vi "Cliente - Fabrica.vi"() -> ()   [LabVIEW 2018]
doc: "Date Client.vi reads the date and time sent from Date Server.vi. The VI first reads 4 bytes defining the length of the date string, then reads the date. Once the stop button is pressed, Date Client sends a single character to tell Date Server to terminate."
uses:
  <vilib>/Utility/file.llb/Write Delimited Spreadsheet (string).vi
panel:
  out "Numeric":dbl
  in  "INICIAR / RESET":bool
  in  "Report:":bool
  in  "RESET \nDE SIMULA敲O":bool
  in  "Emergência":bool
  out "Chave":string
  out "Pedido":string
  out "Pedido":u32(colorbox)
  out "Funcionamento:":string
  out "Funcionamento:":u32(colorbox)
  out "LED Forno":bool
  out "LED Misturador":bool
  out "Protocolo de Comunicação - Produção":string
  out "Estoque \nProduto Final":dbl(slide) scale=0.0..2500.0
  in  "Esteira":bool
  out "Estoque \nForno":dbl(slide) scale=0.0..2000.0
  out "Thermometro\nForno":dbl(slide) scale=0.0..100.0
  in  "Contagem de Estoque OK?":bool
  out "Estoque B utilizado:":dbl
  in  "Estoque A utilizado:":dbl
  out "Estoque \nMisturador":dbl(slide) scale=0.0..2000.0
  in  "Estoque Produto B":dbl min=0.0 max=1000.0
  in  "Estoque Produto A":dbl=1000.0 min=0.0 max=1000.0
  out "Estoque \nProduto B [KG]":dbl(slide) scale=0.0..1200.0
  out "Estoque \nProduto A [KG]":dbl(slide) scale=0.0..1200.0
  out "Protocolo de Ordens de Produção:":string
  in  "Temperatura Desejada Forno °C":dbl(knob) scale=0.0..100.0
  in  "Histórico":i32(listbox)
  out "RESET":dbl
  out "Temperatura Caldeira":dbl
  out "Produto B":dbl
  out "Produto A":dbl
  out "Estado Motor Esteira":dbl
  out "VETOR DE SAIDA":dbl[](array[numeric])
  in  "stop":bool
  out "Mensagem Recebida":string
  in  "Enviar":bool
  in  "Mensagem":string
  in  "Endereço IP":string
  in  "Porta que será utilizada para a conexão":u16=6341
  # "Cliente - Chão de Fábrica"
  # "Comunicação TCP/IP  -  CLIENTE"
  # "Produção Infante Calderaria"
  # "CONTROLE DE ESTOQUE:"
  # "Digite o inventário realizado \ndas matérias - primas abaixo:"
  # "Digite o estoque que será utilizado em produção:"
  # "CONTROLE DE PRODU敲O:"
  # "ORDENS DE PRODU敲O:"
  # "1 - ON ; 0 - OFF"
  # "1 - ON ; 0 - OFF"
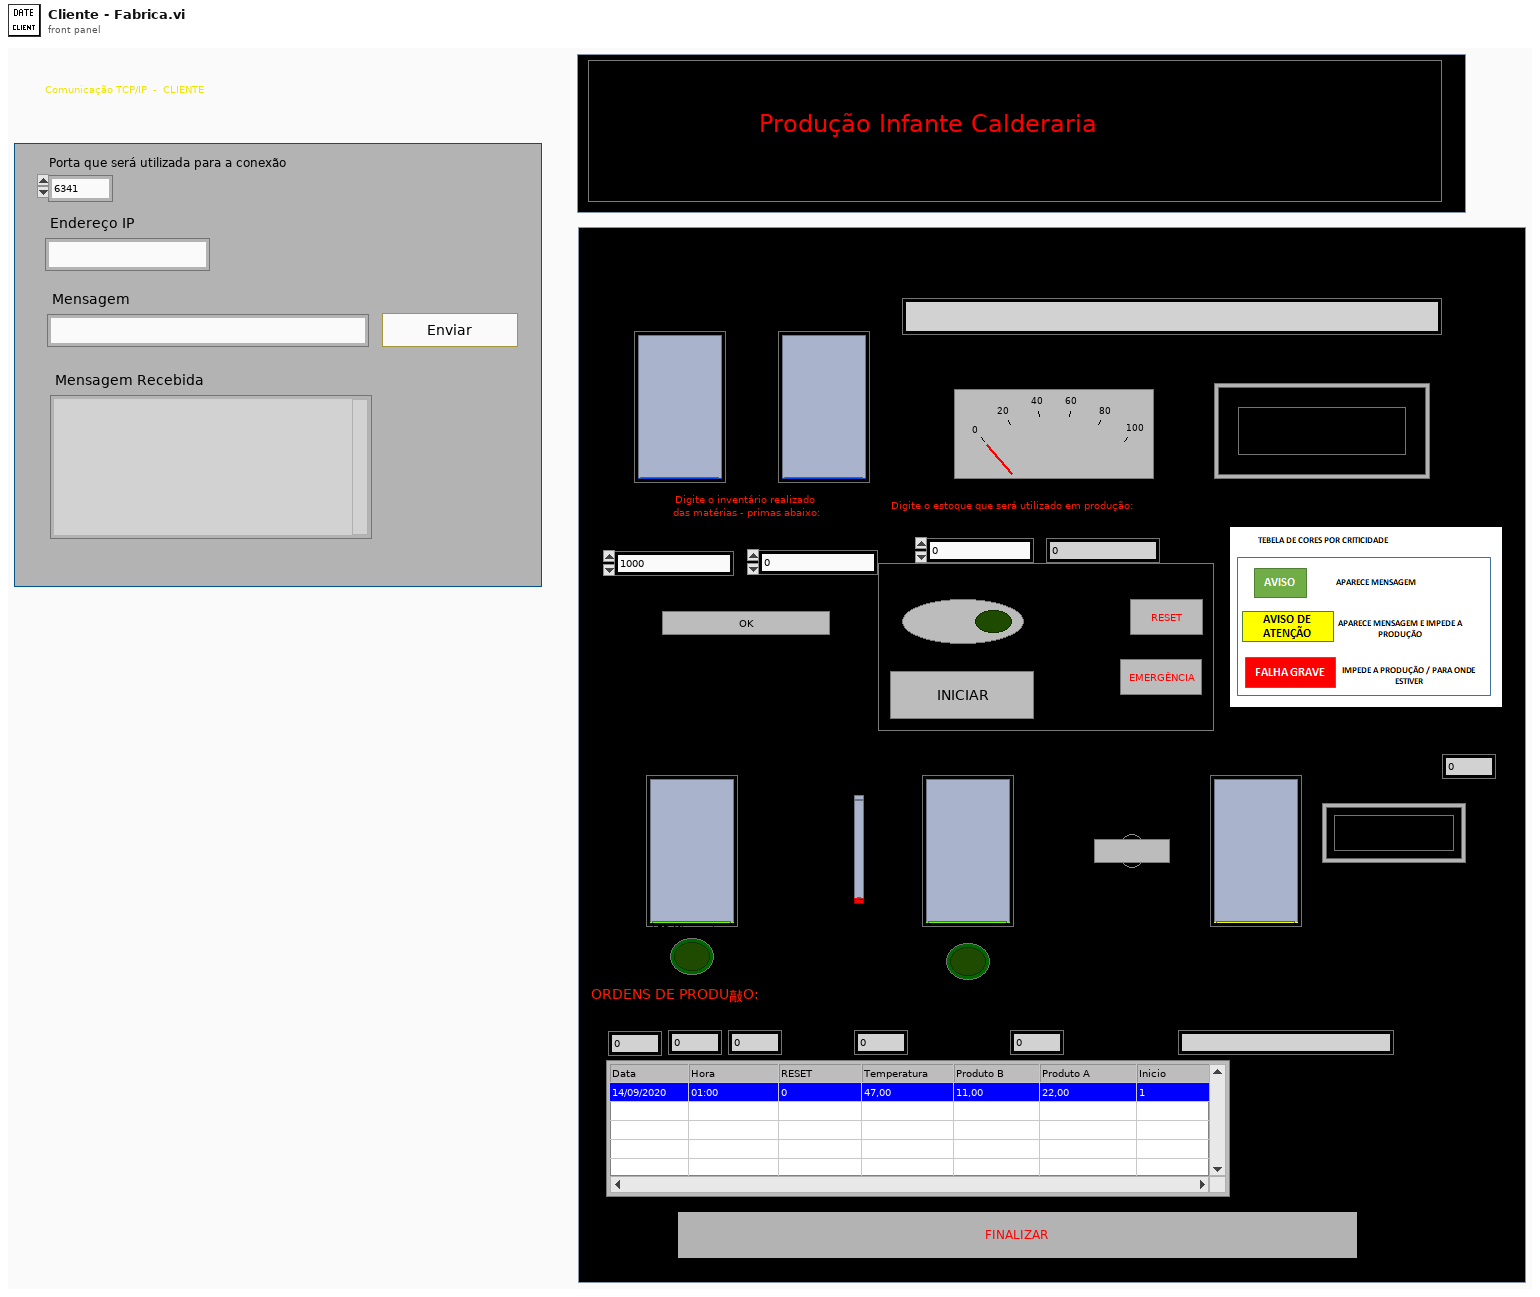
[diagram p1: front panel]
types:
  T1 = enum16{"Standard", "Buffered", "CRLF", "Immediate"}
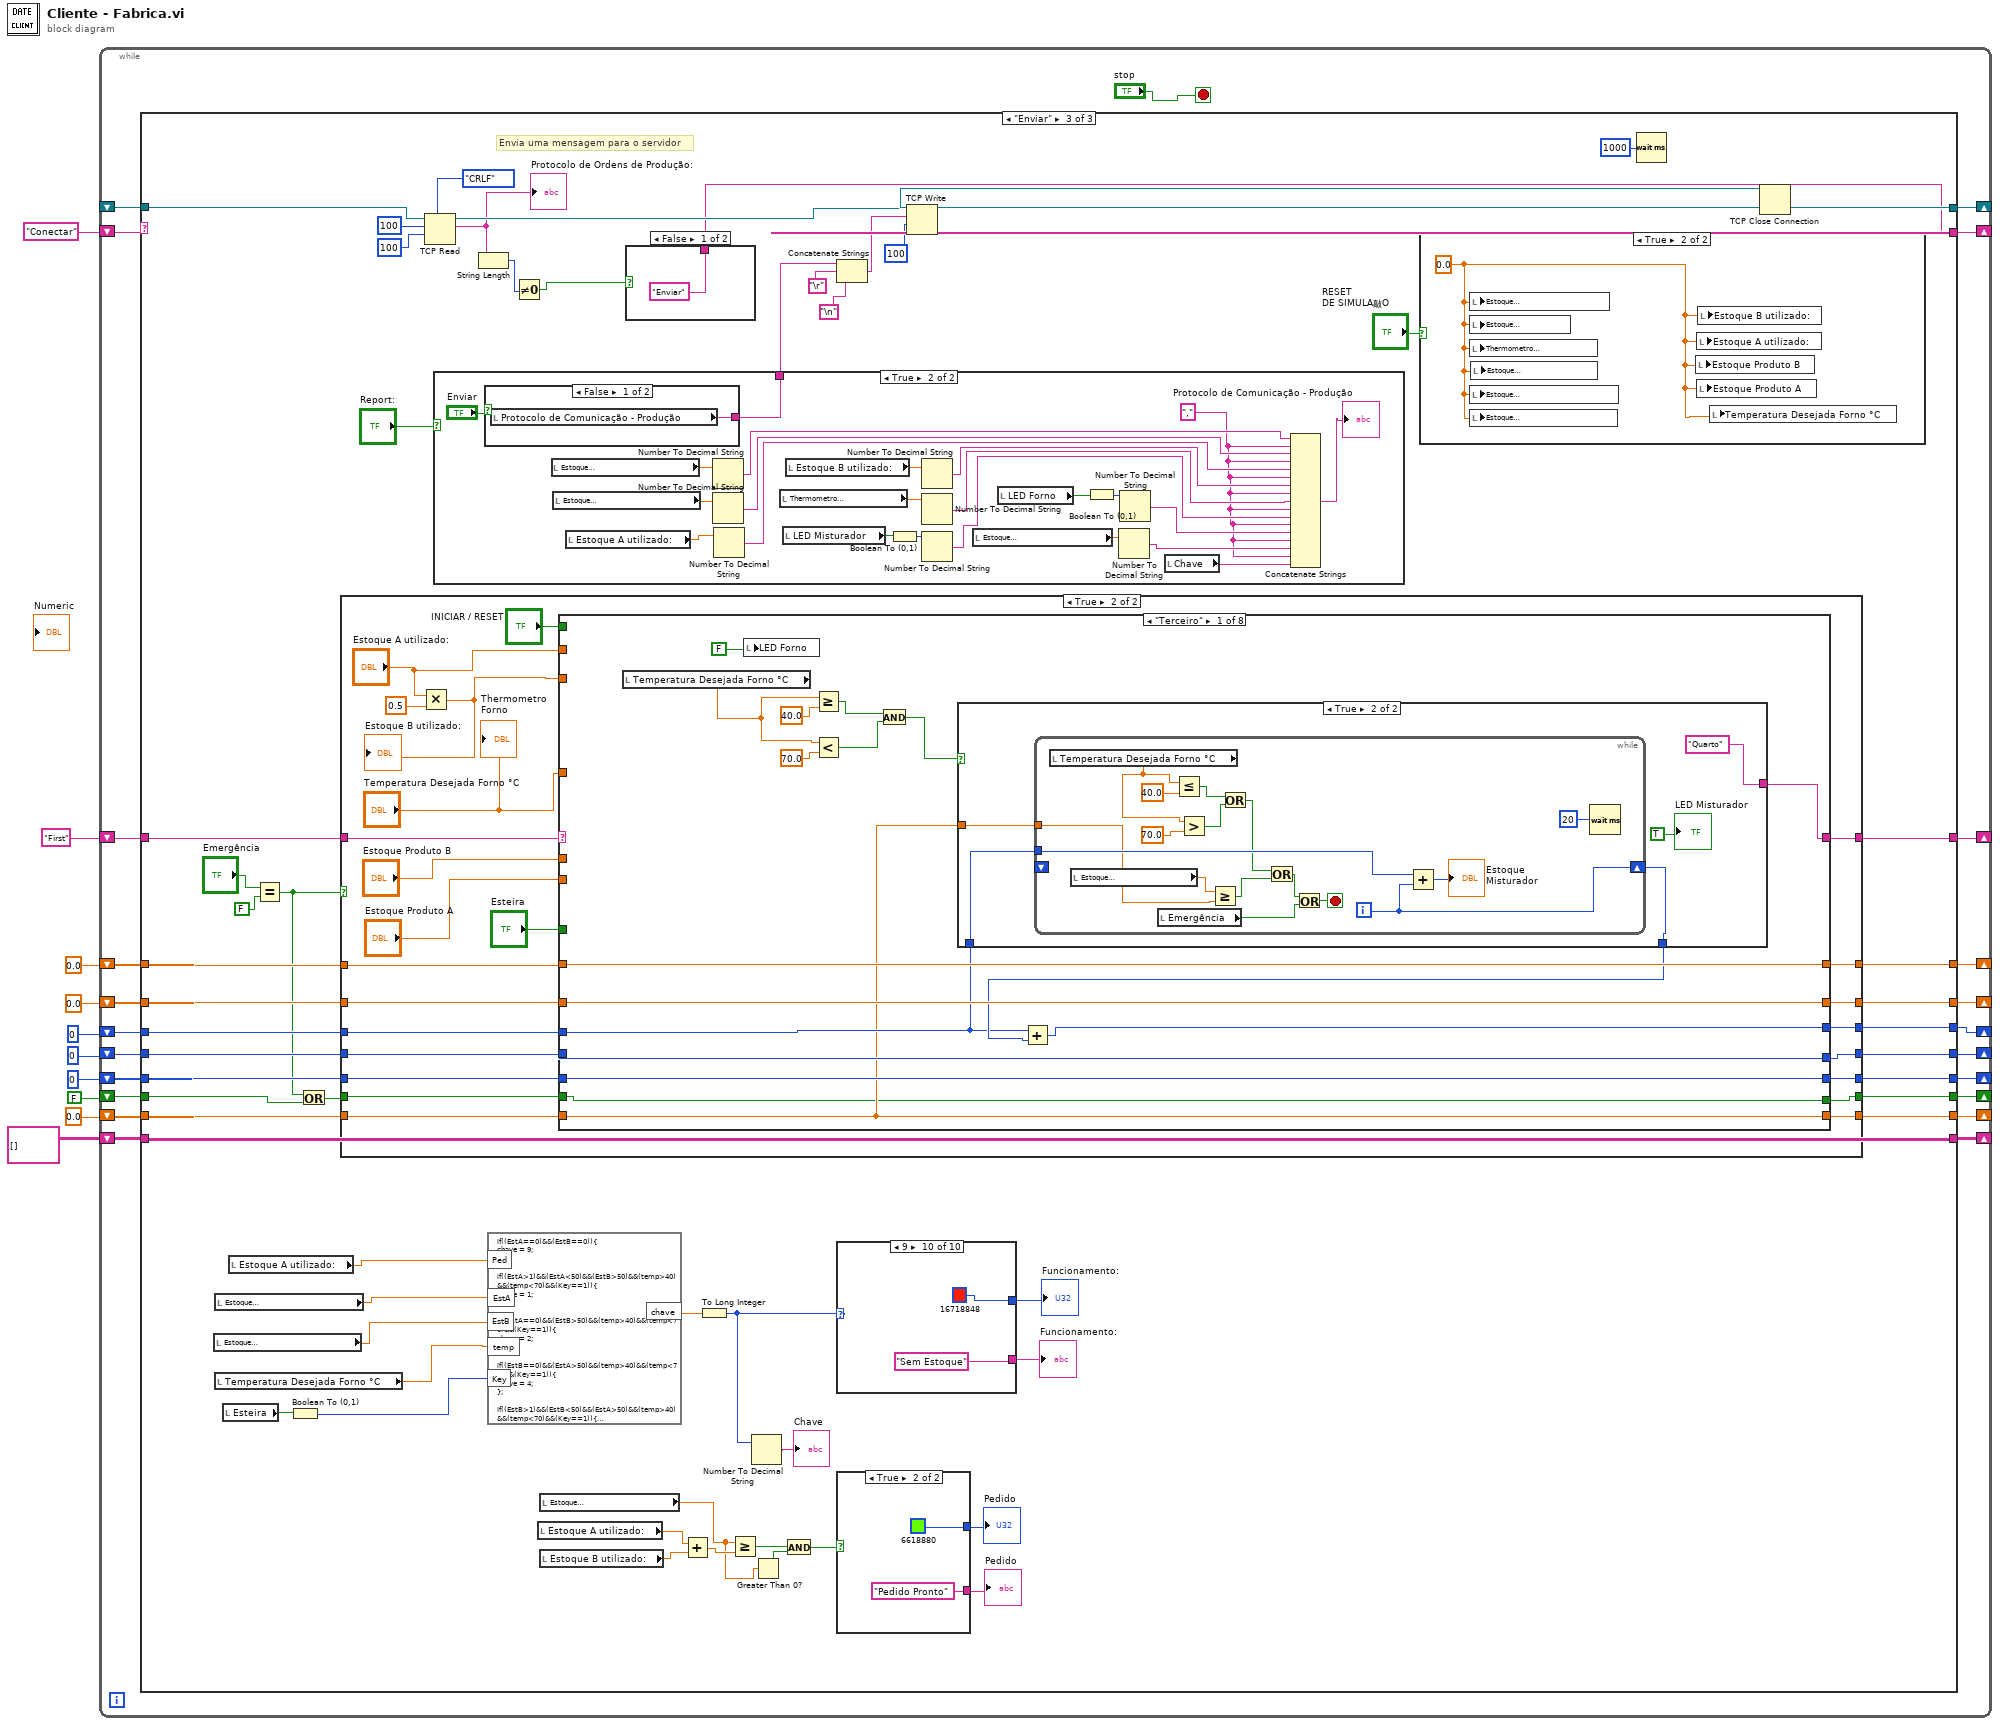
[diagram p0: block diagram]
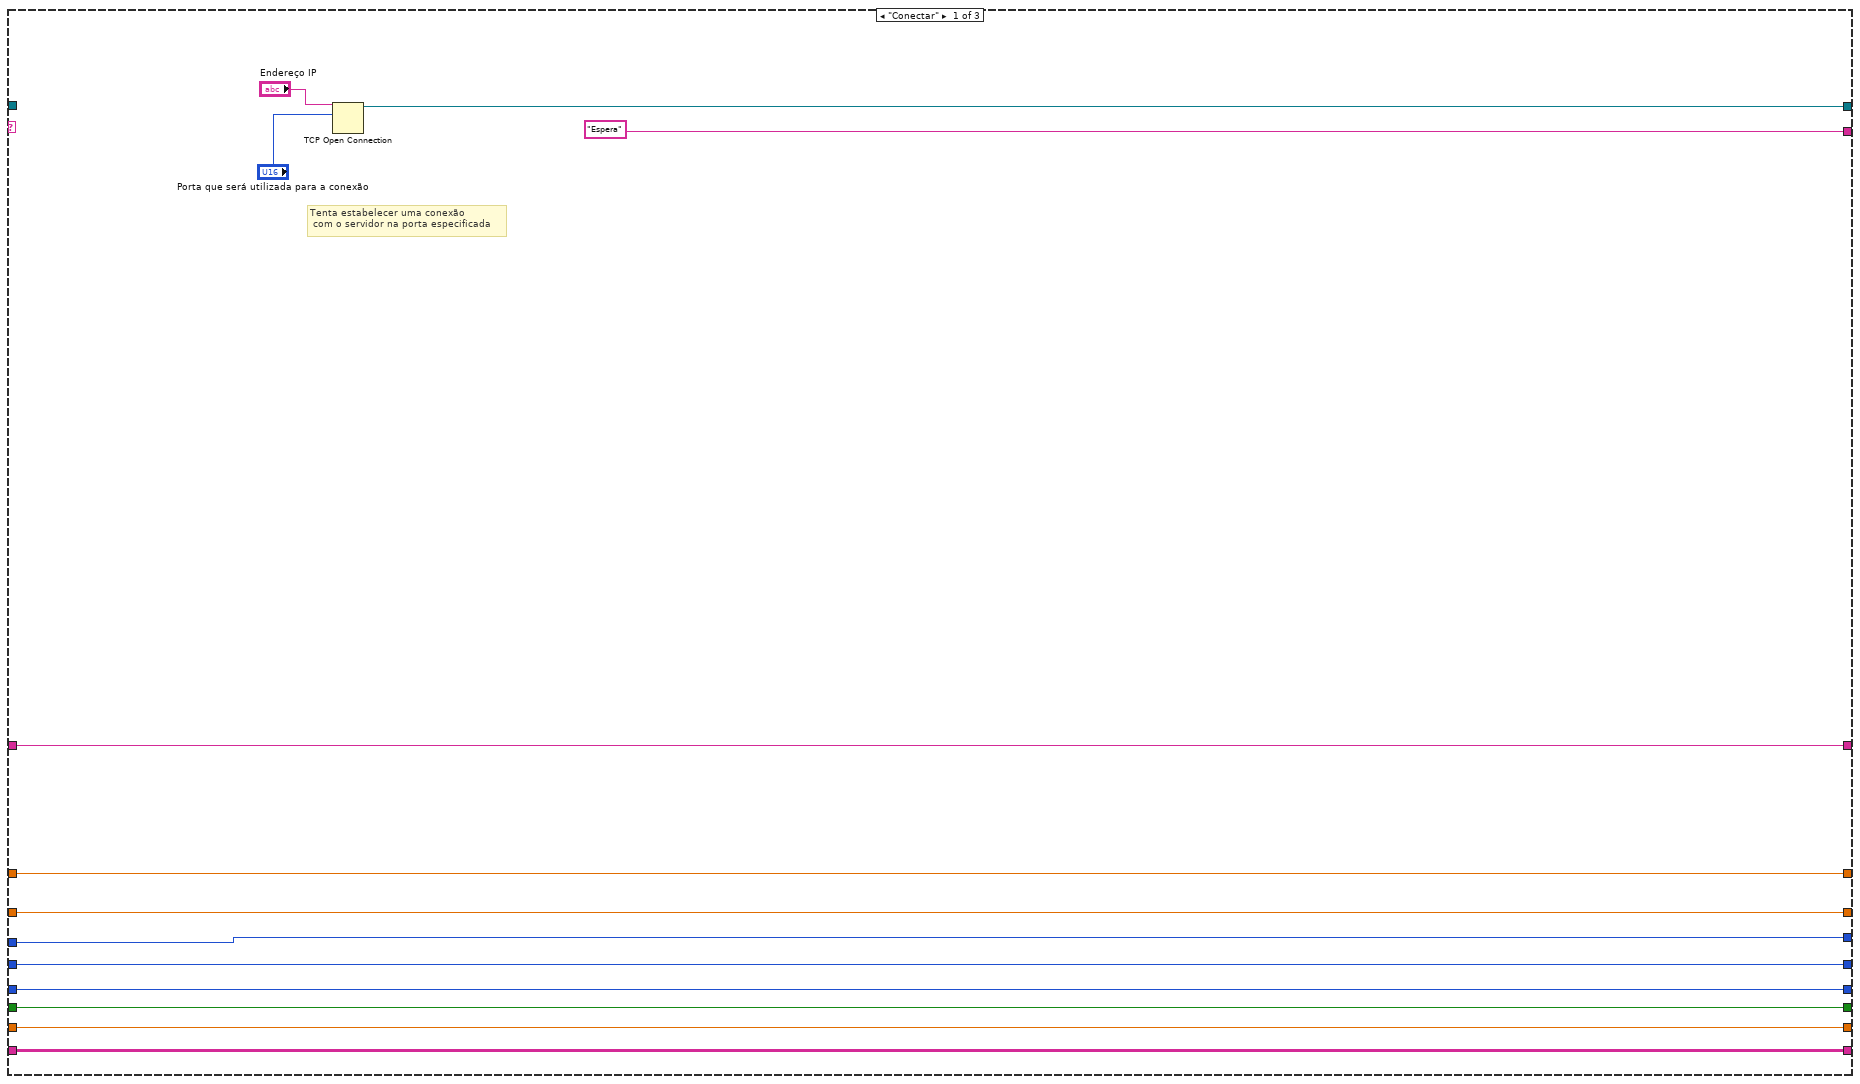
[diagram p2: hidden frame]
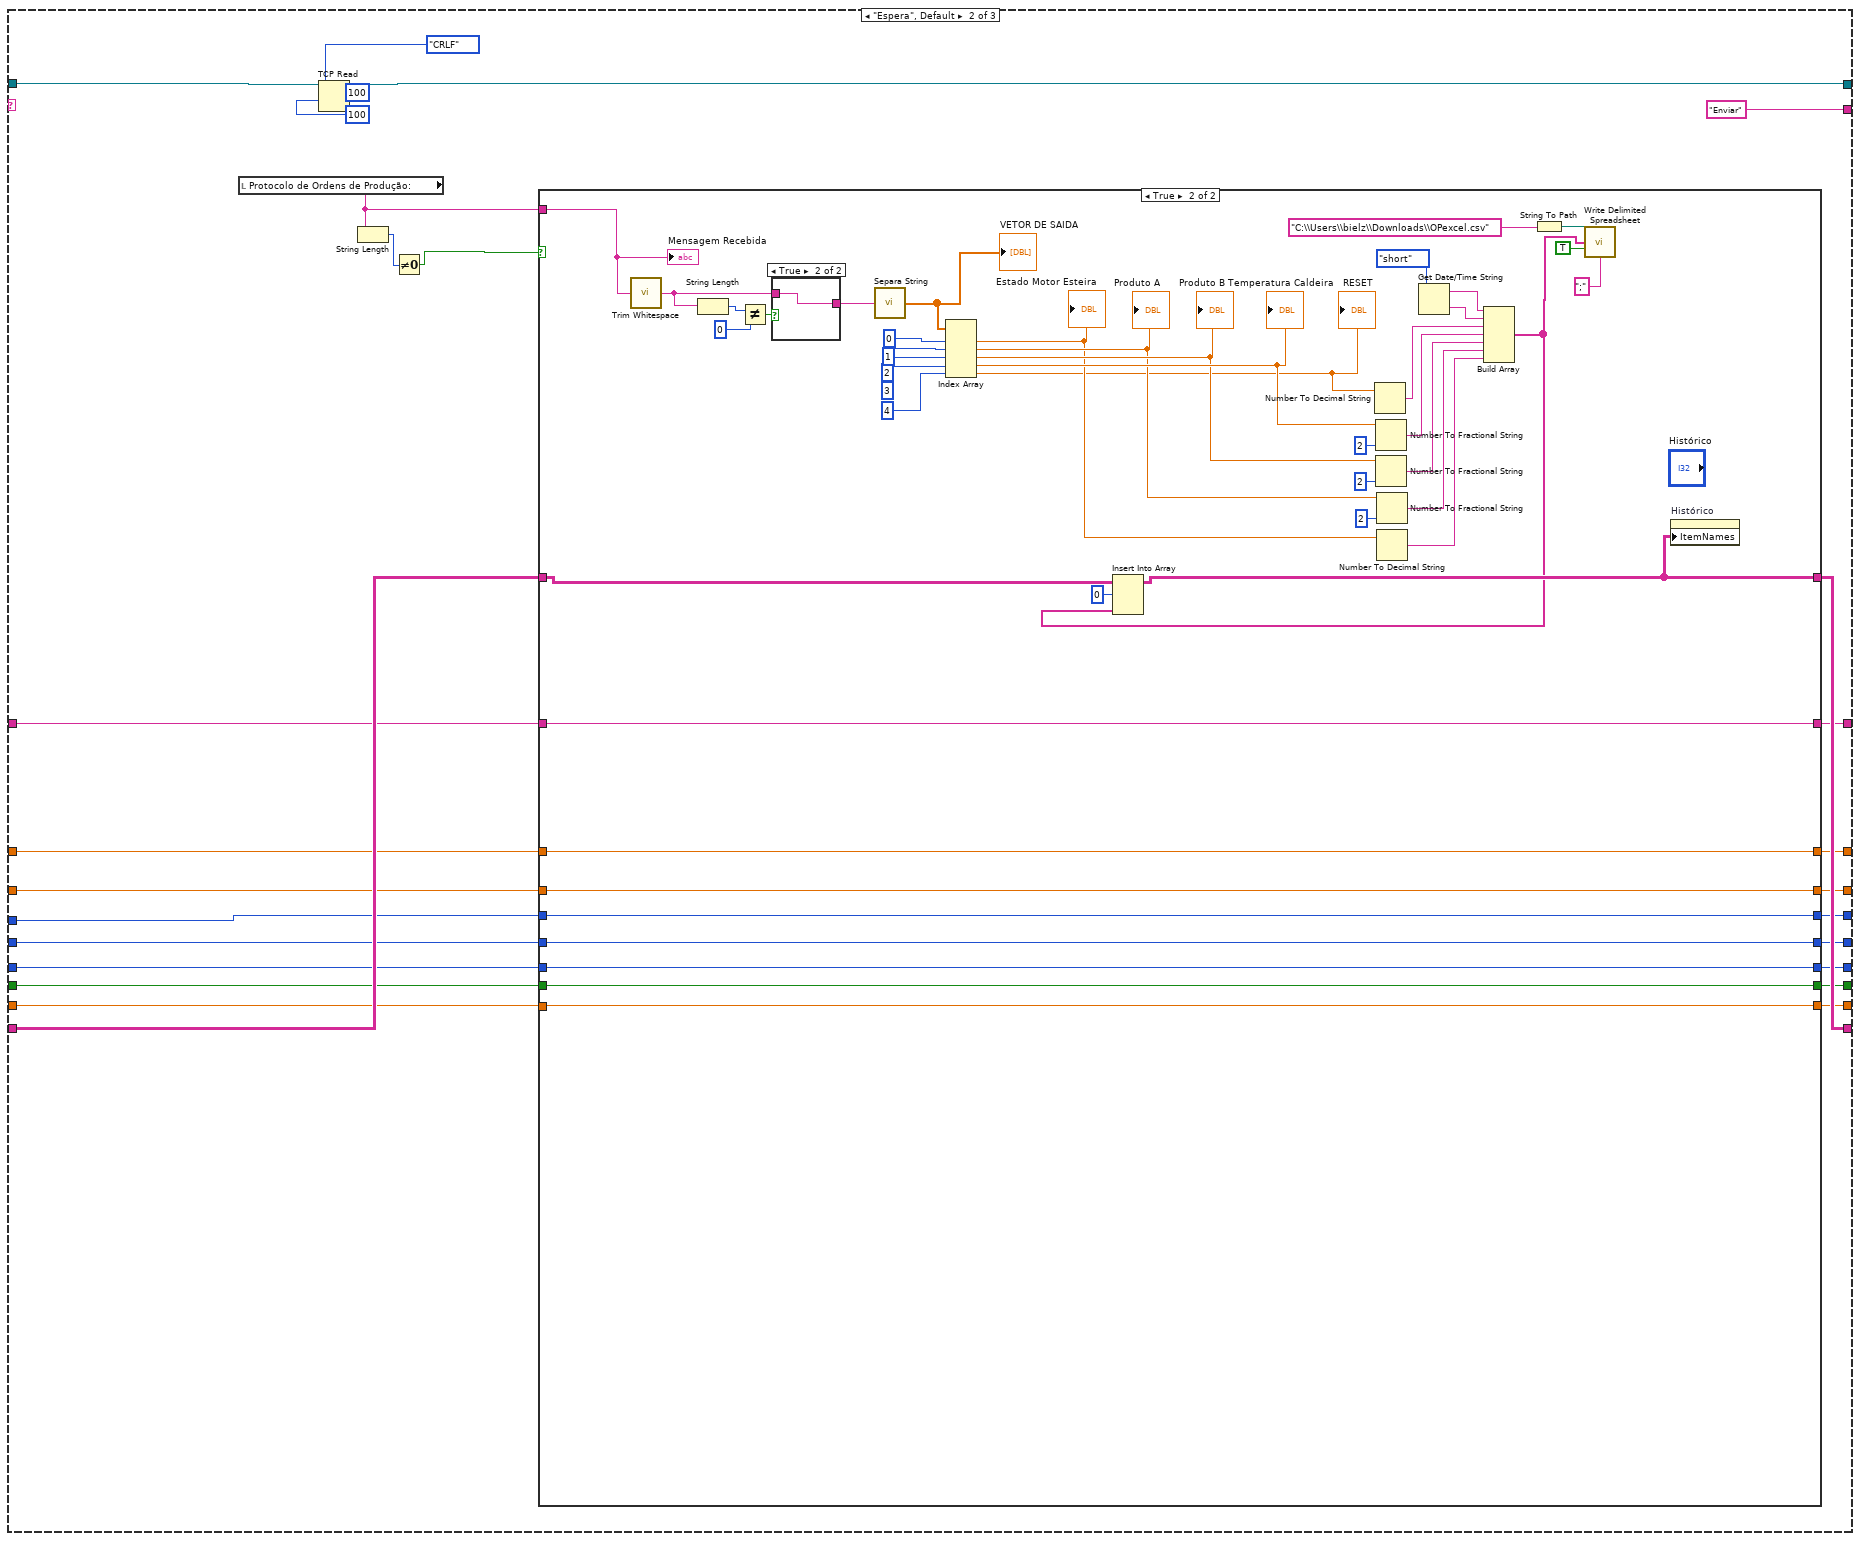
[diagram p3: hidden frame]
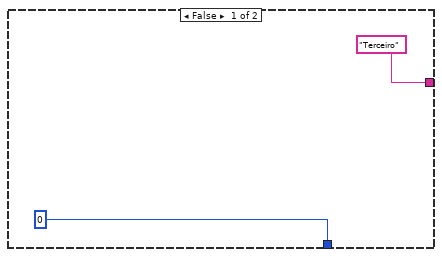
[diagram p7: hidden frame]
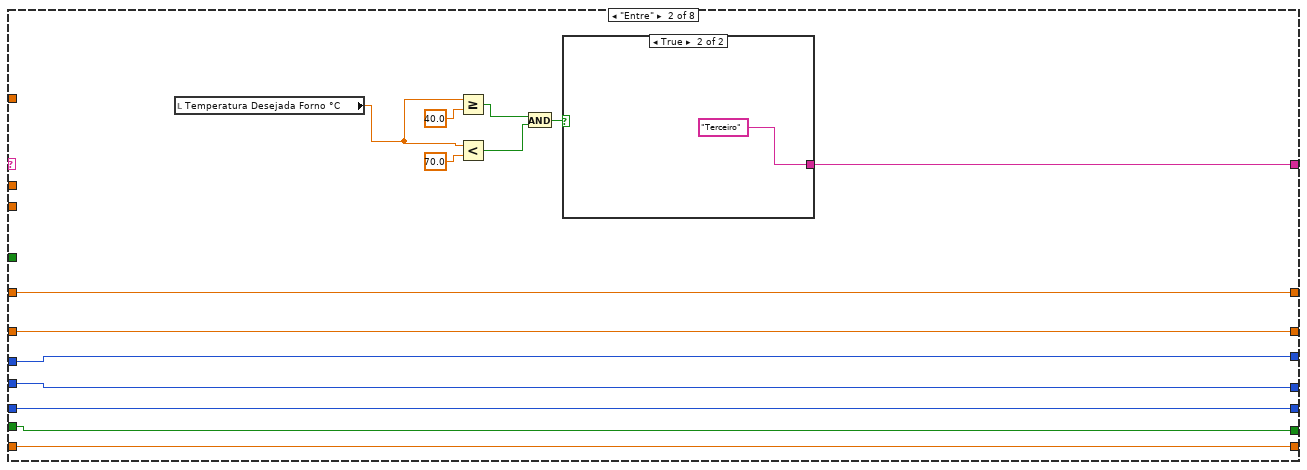
[diagram p8: hidden frame]
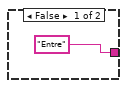
[diagram p9: hidden frame]
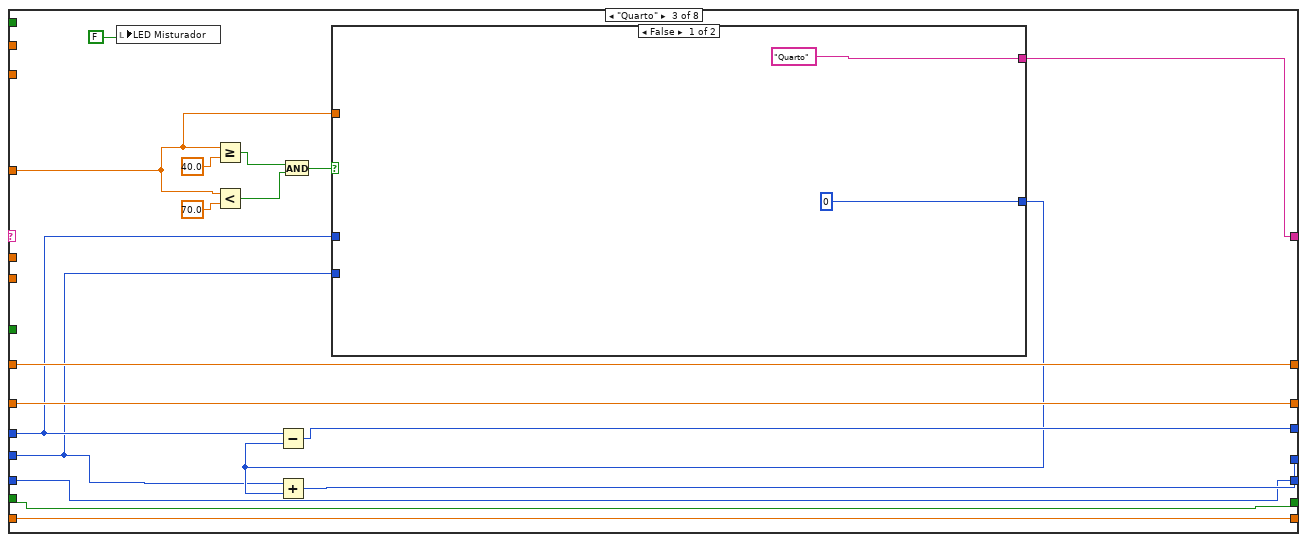
[diagram p10: hidden frame]
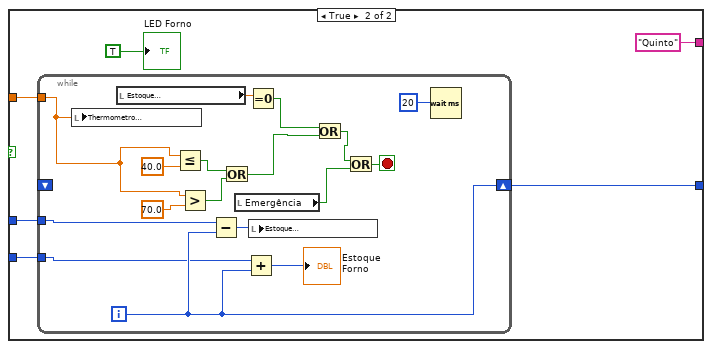
[diagram p11: hidden frame]
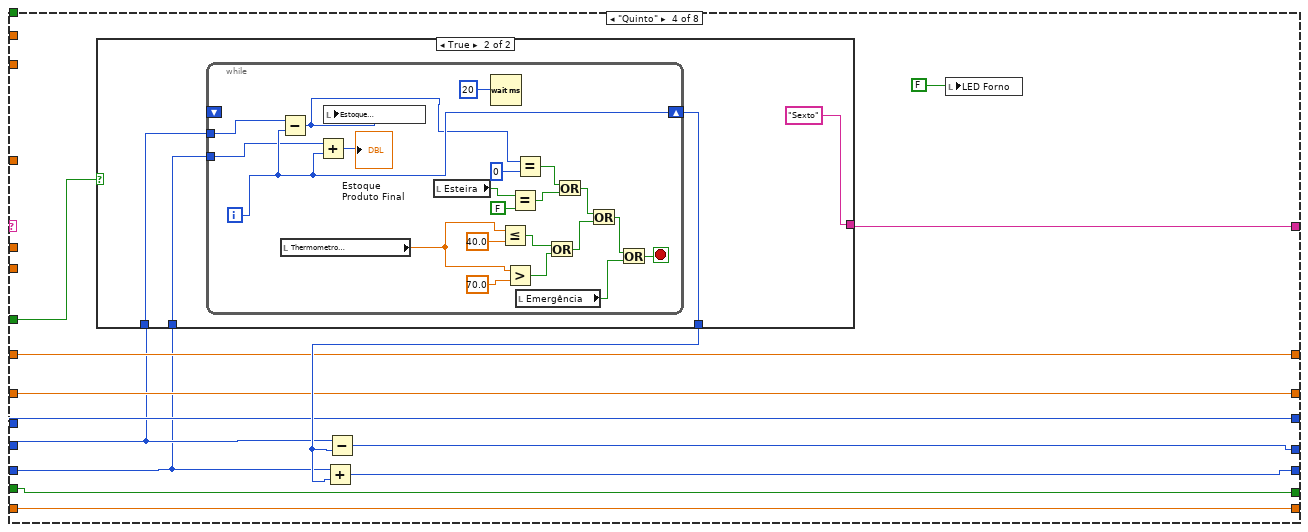
[diagram p12: hidden frame]
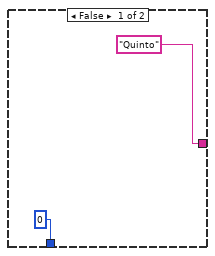
[diagram p13: hidden frame]
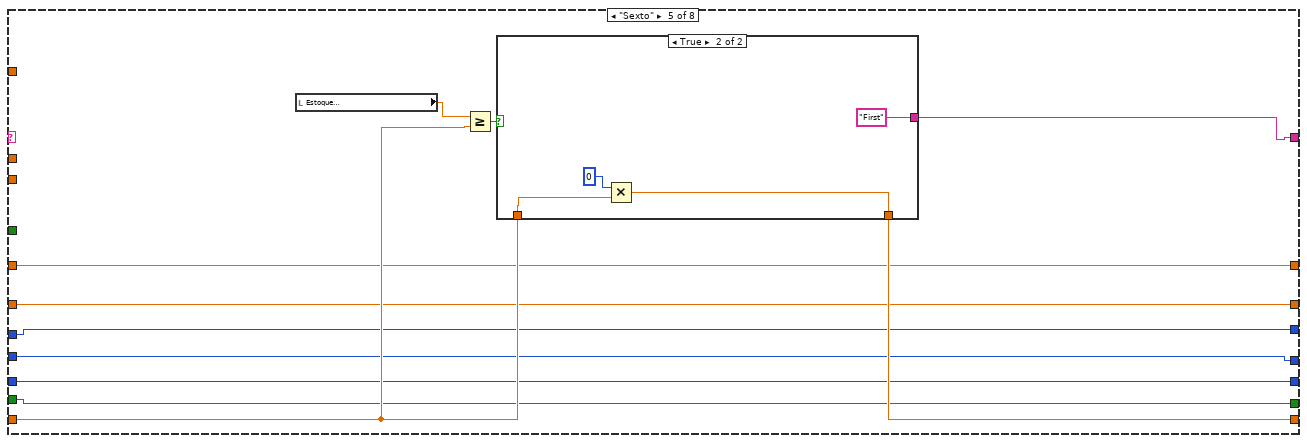
[diagram p14: hidden frame]
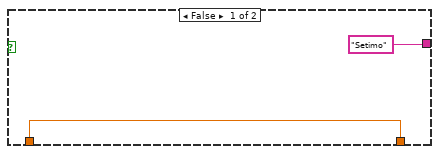
[diagram p15: hidden frame]
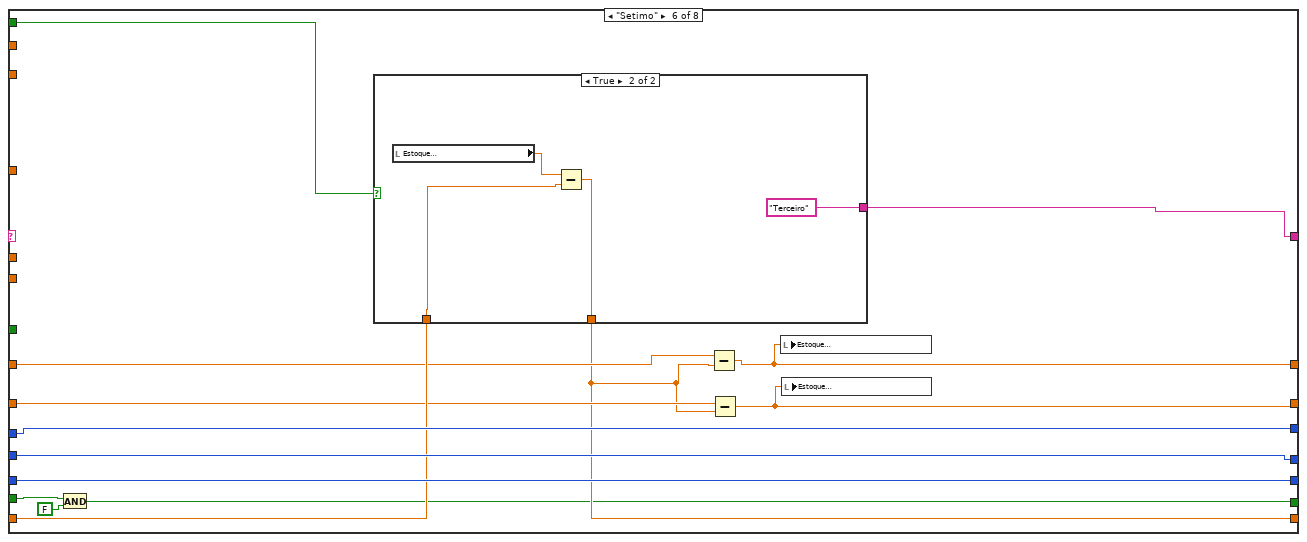
[diagram p16: hidden frame]
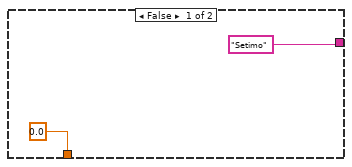
[diagram p17: hidden frame]
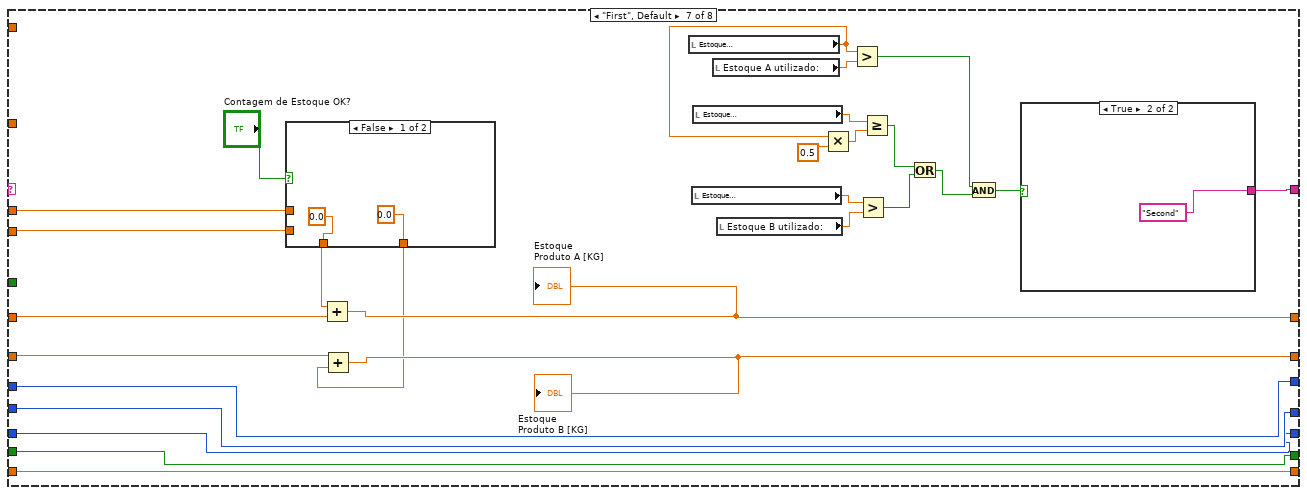
[diagram p18: hidden frame]
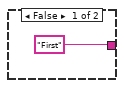
[diagram p19: hidden frame]
diagram:
  n1 = while {
    shift-right: [w33] -> _
    shift-left: "Conectar" -> [w34]
    shift-right: [w28] -> w10
    shift-left: _ -> [w29]
    shift-right: [w31] -> _
    shift-left: string[][] [] -> [w30]
    shift-right: [w26] -> _
    shift-left: "First" -> [w27]
    shift-right: [w23] -> _
    shift-left: 0.0 -> [w24]
    shift-right: [w22] -> _
    shift-left: 0.0 -> [w25]
    shift-right: [w20] -> _
    shift-left: 0 -> [w21]
    shift-right: [w18] -> _
    shift-left: 0 -> [w19]
    shift-right: [w16] -> _
    shift-left: 0 -> [w17]
    shift-right: [w14] -> _
    shift-left: 0.0 -> [w15]
    shift-right: [w12] -> _
    shift-left: FALSE -> [w13]
    stop <- "stop" stop-if-true
    n2 = case shown="\"Enviar\"" w34 {
      tunnel: [w43 w70 w187] -> w28
      tunnel: ["Espera" "Enviar" w174] -> w33
      tunnel: w29 -> [_ w66 w172]
      tunnel: [w44 w68 w181] -> w31
      tunnel: w30 -> [w44 w67 w181]
      tunnel: w27 -> [w41 w59 w139]
      tunnel: [w41 w60 w170] -> w26
      tunnel: w25 -> [w40 w61 w169]
      tunnel: w24 -> [w42 w63 w168]
      tunnel: [w42 w64 w167] -> w23
      tunnel: [w40 w62 w166] -> w22
      tunnel: w21 -> [w39 w58 w164]
      tunnel: [w39 w57 w163] -> w20
      tunnel: w19 -> [w38 w55 w162]
      tunnel: [w38 w56 w160] -> w18
      tunnel: w17 -> [w37 w54 w161]
      tunnel: [w37 w53 w159] -> w16
      tunnel: w15 -> [w36 w50 w138]
      tunnel: [w36 w51 w137] -> w14
      tunnel: w13 -> [w35 w48 w129]
      tunnel: [w35 w49 w132] -> w12
      frame "Conectar" {
        # "Tenta estabelecer uma conexão\n com o servidor na porta especificada"
        n3 = TCP Open Connection(address="Endereço IP", remote port or service name="Porta que será utilizada para a conexão") -> (connection ID=w43:refnum<k5>)  [unwired: 3 in, 1 out]
      }
      frame "Espera", Default {
        n4 = local read "Protocolo de Ordens de Produção:"() -> (w65:string)
        n5 = TCP Read(connection ID=w66, bytes to read=100, 7:T1."CRLF" ("mode (standard)"), 9:100 ("timeout ms (25000)")) -> (connection ID out=w70:refnum<k5>)  [unwired: 1 in, 2 out]
        n6 = String Length(string=w65) -> (length=w72:i32)
        n7 = Not Equal To 0?(x=w72) -> (x != 0?=w71:bool)
        n8 = case shown="True" w71 {
          tunnel: w65 -> [_ w127]
          tunnel: [w83 w106] -> w68
          tunnel: w67 -> [w83 w116]
          tunnel: [w82 w91] -> w64
          tunnel: w63 -> [w82 w91]
          tunnel: [w81 w90] -> w62
          tunnel: w61 -> [w81 w90]
          tunnel: [w80 w89] -> w60
          tunnel: w59 -> [w80 w89]
          tunnel: w58 -> [w79 w88]
          tunnel: [w79 w88] -> w57
          tunnel: w55 -> [w78 w87]
          tunnel: [w78 w87] -> w56
          tunnel: w54 -> [w77 w86]
          tunnel: [w77 w86] -> w53
          tunnel: w50 -> [w76 w85]
          tunnel: [w76 w85] -> w51
          tunnel: [w75 w84] -> w49
          tunnel: w48 -> [w75 w84]
          frame False {
          }
          frame True {
            n9 = call <vilib>:"Trim Whitespace.vi"("string"=w127) -> ("trimmed string"=w102:string)  [unwired: 1 in]
            n10 = String Length(string=w102) -> (length=w101:i32)
            n11 = Not Equal?(x=w101, y=0) -> (x != y?=w104:bool)
            n12 = case shown="True" w104 {
              tunnel: [_ w128] -> w103
              tunnel: w102 -> [_ w128]
              frame False {
              }
              frame True {
              }
            }
            n13 = call "Separa String.vi"("TEXTO DE ENTRADA"=w103) -> ("VETOR DE SAIDA"=w122:dbl[])
            "VETOR DE SAIDA" <- w122
            n14 = Index Array(array=w122, index #1=0 ("index"), index #2=1 ("index"), index #3=2 ("index"), index #4=3 ("index"), index #5=4 ("index")) -> (element #1=w98:dbl, element #2=w110:dbl, element #3=w111:dbl, element #4=w112:dbl, element #5=w95:dbl)
            "Estado Motor Esteira" <- w98
            "Produto A" <- w110
            "Produto B" <- w111
            "Temperatura Caldeira" <- w112
            "RESET" <- w95
            n15 = Number To Decimal String(number=w95) -> (decimal integer string=w96:string)  [unwired: 1 in]
            n16 = Number To Fractional String(number=w112, precision (6)=i16 2) -> (F-format string=w109:string)  [unwired: 2 in]
            n17 = Number To Fractional String(number=w111, precision (6)=i16 2) -> (F-format string=w108:string)  [unwired: 2 in]
            n18 = Number To Fractional String(number=w110, precision (6)=i16 2) -> (F-format string=w107:string)  [unwired: 2 in]
            n19 = Number To Decimal String(number=w98) -> (decimal integer string=w97:string)  [unwired: 1 in]
            n20 = Get Date/Time String(date format (0)=enum16{"short", "long", "abbreviated"}."short") -> (date string=w93:string, time string=w94:string)  [unwired: 2 in]
            n21 = Build Array(w93, w94, w96, w109, w108, w107, w97) -> (w105:string[])
            n22 = Insert Into Array(array=w116, index (row)=0 ("index"), new element=w105) -> (w106:string[][])  [unwired: 1 in]
            n23 = String To Path(string="C:\\Users\\bielz\\Downloads\\OPexcel.csv") -> (path=w118:path)
            n24 = call-poly <vilib>:"Write Delimited Spreadsheet.vi"("file path (dialog if empty)"=w118, "1D data"=w105, "append to file? (new file:F)"=TRUE, "delimiter (\\t)"=";") -> ()  [unwired: 10 in, 2 out]
            n25 = property on="Histórico" class="MCListbox (strict)"("ItemNames"=w106) -> ()  [unwired: 2 in, 2 out]
            "Mensagem Recebida" <- w127
          }
        }
      }
      frame "Enviar" {
        # "Envia uma mensagem para o servidor"
        n26 = local read "Estoque \nProduto B [KG]"() -> (w156:dbl)
        n27 = local read "Estoque \nProduto A [KG]"() -> (w157:dbl)
        n28 = local read "Temperatura Desejada Forno °C"() -> (w155:dbl)
        n29 = local read "Esteira"() -> (w154:bool)
        n30 = local read "Estoque A utilizado:"() -> (w140:dbl)
        n31 = Equal?(x="Emergência", y=FALSE) -> (x = y?=w130:bool)
        n32 = Boolean To (0,1)(Boolean=w154) -> (0, 1=w153:i16)
        n33 = Or(x=w130, y=w129) -> (x .or. y?=w131:bool)
        n34 = case shown="True" w130 {
          tunnel: [w192 w219] -> w170
          tunnel: w169 -> [w194 w218]
          tunnel: w168 -> [w195 w217]
          tunnel: [w195 w216] -> w167
          tunnel: [w194 w215] -> w166
          tunnel: w164 -> [w191 w212]
          tunnel: [w191 w211] -> w163
          tunnel: w162 -> [w190 w210]
          tunnel: w161 -> [w189 w209]
          tunnel: [w190 w208] -> w160
          tunnel: [w189 w207] -> w159
          tunnel: w139 -> [w192 w204]
          tunnel: w138 -> [w193 w200]
          tunnel: [w193 w199] -> w137
          tunnel: w131 -> [w188 w197]
          tunnel: [w188 w196] -> w132
          frame False {
          }
          frame True {
            n35 = Multiply(x="Estoque A utilizado:", y=0.5) -> (x*y=w203:dbl)
            "Estoque B utilizado:" <- w203
            n36 = case shown="\"Terceiro\"" w204 {
              tunnel: [w226 w268 w278 w320 w368 w381 w416 w442] -> w219
              tunnel: w218 -> [w236 w270 w290 w327 w361 w384 w421 w447]
              tunnel: w217 -> [w235 w269 w291 w326 w360 w385 w422 w440]
              tunnel: [w235 w269 w291 w326 w360 w383 w420 w446] -> w216
              tunnel: [w236 w270 w290 w327 w361 w382 w419 w445] -> w215
              tunnel: "Estoque A utilizado:" -> [_ _ _ _ _ _ _ w435]
              tunnel: "Estoque Produto A" -> [_ _ _ _ _ _ w415 _]
              tunnel: "Estoque Produto B" -> [_ _ _ _ _ _ w414 _]
              tunnel: w212 -> [w223 w271 w286 w328 w362 w387 w412 w438]
              tunnel: [w234 w271 w292 w328 w362 w387 w412 w438] -> w211
              tunnel: w210 -> [w233 w272 w285 w325 w363 w388 w406 w437]
              tunnel: [w233 w272 w293 w329 w363 w388 w406 w437] -> w208
              tunnel: w209 -> [w232 w273 w289 w324 w364 w389 w405 w436]
              tunnel: [w232 w273 w289 w330 w364 w389 w405 w436] -> w207
              tunnel: w203 -> [_ _ _ _ _ _ _ w434]
              tunnel: "Esteira" -> [_ _ _ w322 _ _ _ _]
              tunnel: "Temperatura Desejada Forno °C" -> [_ _ w279 _ _ _ _ _]
              tunnel: w200 -> [w221 w261 w277 w321 w366 w386 w397 w432]
              tunnel: [w221 w261 w277 w321 w369 w380 w397 w430] -> w199
              tunnel: "INICIAR / RESET" -> [_ _ _ _ _ w379 _ w433]
              tunnel: w197 -> [w220 w260 w276 w319 w359 w377 w396 w429]
              tunnel: [w220 w260 w276 w319 w359 w376 w396 w429] -> w196
              frame "Terceiro" {
                n37 = local read "Temperatura Desejada Forno °C"() -> (w222:dbl)
                n38 = local write "LED Forno"(FALSE) -> ()
                n39 = Greater Or Equal?(x=w222, y=40.0) -> (x >= y?=w229:bool)
                n40 = Less?(x=w222, y=70.0) -> (x < y?=w227:bool)
                n41 = And(x=w229, y=w227) -> (x .and. y?=w225:bool)
                n42 = case shown="True" w225 {
                  tunnel: ["Terceiro" "Quarto"] -> w226
                  tunnel: [0 w242] -> w224
                  tunnel: w223 -> [_ w241]
                  tunnel: w221 -> [_ w240]
                  frame False {
                  }
                  frame True {
                    n43 = while {
                      shift-right: [w257] -> w242
                      shift-left: _ -> [_]
                      tunnel: w241 -> [w256]
                      tunnel: w240 -> [w248]
                      i -> [w257]
                      stop <- w246 stop-if-true
                      n44 = local read "Temperatura Desejada Forno °C"() -> (w250:dbl)
                      n45 = local read "Estoque \nMisturador"() -> (w247:dbl)
                      n46 = local read "Emergência"() -> (w245:bool)
                      n47 = Less Or Equal?(x=w250, y=40.0) -> (x <= y?=w253:bool)
                      n48 = Greater?(x=w250, y=70.0) -> (0:w252:bool)
                      n49 = Greater Or Equal?(x=w247, y=w248) -> (x >= y?=w249:bool)
                      n50 = Or(x=w253, y=w252) -> (x .or. y?=w251:bool)
                      n51 = Or(x=w251, y=w249) -> (x .or. y?=w244:bool)
                      n52 = Or(x=w244, y=w245) -> (x .or. y?=w246:bool)
                      n53 = Add(x=w256, y=w257) -> (x+y=→"Estoque \nMisturador":i32)
                      n54 = Wait (ms)(milliseconds to wait=20) -> ()  [unwired: 1 out]
                    }
                    "LED Misturador" <- TRUE
                  }
                }
                n55 = Add(x=w223, y=w224) -> (x+y=w234:i32)
              }
              frame "Entre" {
                n56 = local read "Temperatura Desejada Forno °C"() -> (w262:dbl)
                n57 = Greater Or Equal?(x=w262, y=40.0) -> (x >= y?=w265:bool)
                n58 = Less?(x=w262, y=70.0) -> (x < y?=w263:bool)
                n59 = And(x=w265, y=w263) -> (x .and. y?=w267:bool)
                n60 = case shown="True" w267 {
                  tunnel: ["Entre" "Terceiro"] -> w268
                  frame False {
                  }
                  frame True {
                  }
                }
              }
              frame "Quarto" {
                n61 = local write "LED Misturador"(FALSE) -> ()
                n62 = Greater Or Equal?(x=w279, y=40.0) -> (x >= y?=w283:bool)
                n63 = Less?(x=w279, y=70.0) -> (x < y?=w281:bool)
                n64 = And(x=w283, y=w281) -> (x .and. y?=w280:bool)
                n65 = case shown="False" w280 {
                  tunnel: [0 w301] -> w287
                  tunnel: w286 -> [_ w300]
                  tunnel: w285 -> [_ w299]
                  tunnel: w279 -> [_ w297]
                  tunnel: ["Quarto" "Quinto"] -> w278
                  frame False {
                  }
                  frame True {
                    n66 = while {
                      shift-right: [w315] -> w301
                      shift-left: _ -> [_]
                      tunnel: w300 -> [w314]
                      tunnel: w299 -> [w313]
                      tunnel: w297 -> [w306]
                      i -> [w315]
                      stop <- w304 stop-if-true
                      n67 = local write "Thermometro\nForno"(w306) -> ()
                      n68 = local read "Estoque \nMisturador"() -> (w318:dbl)
                      n69 = Less Or Equal?(x=w306, y=40.0) -> (x <= y?=w308:bool)
                      n70 = Greater?(x=w306, y=70.0) -> (0:w307:bool)
                      n71 = Subtract(x=w314, y=w315) -> (x-y=w312:i32)
                      n72 = Or(x=w308, y=w307) -> (x .or. y?=w305:bool)
                      n73 = local read "Emergência"() -> (w303:bool)
                      n74 = Add(x=w313, y=w315) -> (x+y=→"Estoque \nForno":i32)
                      n75 = Equal To 0?(x=w318) -> (x = 0?=w317:bool)
                      n76 = local write "Estoque \nMisturador"(w312) -> ()
                      n77 = Or(x=w317, y=w305) -> (x .or. y?=w302:bool)
                      n78 = Or(x=w302, y=w303) -> (x .or. y?=w304:bool)
                      n79 = Wait (ms)(milliseconds to wait=20) -> ()  [unwired: 1 out]
                    }
                    "LED Forno" <- TRUE
                  }
                }
                n80 = Subtract(x=w286, y=w287) -> (x-y=w292:i32)
                n81 = Add(x=w285, y=w287) -> (x+y=w293:i32)
              }
              frame "Quinto" {
                n82 = case shown="True" w322 {
                  tunnel: [0 w337] -> w331
                  tunnel: w325 -> [_ w336]
                  tunnel: w324 -> [_ w335]
                  tunnel: ["Quinto" "Sexto"] -> w320
                  frame False {
                  }
                  frame True {
                    n83 = while {
                      shift-right: [w355] -> w337
                      shift-left: _ -> [_]
                      tunnel: w336 -> [w354]
                      tunnel: w335 -> [w353]
                      i -> [w355]
                      stop <- w340 stop-if-true
                      n84 = Subtract(x=w354, y=w355) -> (x-y=w348:i32)
                      n85 = local read "Thermometro\nForno"() -> (w344:dbl)
                      n86 = Add(x=w353, y=w355) -> (x+y=→"Estoque \nProduto Final":i32)
                      n87 = local write "Estoque \nForno"(w348) -> ()
                      n88 = local read "Esteira"() -> (w356:bool)
                      n89 = Wait (ms)(milliseconds to wait=20) -> ()  [unwired: 1 out]
                      n90 = Less Or Equal?(x=w344, y=40.0) -> (x <= y?=w346:bool)
                      n91 = Greater?(x=w344, y=70.0) -> (0:w345:bool)
                      n92 = Equal?(x=w356, y=FALSE) -> (x = y?=w351:bool)
                      n93 = Equal?(x=w348, y=0) -> (x = y?=w349:bool)
                      n94 = local read "Emergência"() -> (w338:bool)
                      n95 = Or(x=w346, y=w345) -> (x .or. y?=w343:bool)
                      n96 = Or(x=w349, y=w351) -> (x .or. y?=w342:bool)
                      n97 = Or(x=w342, y=w343) -> (x .or. y?=w339:bool)
                      n98 = Or(x=w339, y=w338) -> (x .or. y?=w340:bool)
                    }
                  }
                }
                n99 = Add(x=w324, y=w331) -> (x+y=w330:i32)
                n100 = Subtract(x=w325, y=w331) -> (x-y=w329:i32)
                n101 = local write "LED Forno"(FALSE) -> ()
              }
              frame "Sexto" {
                n102 = local read "Estoque \nProduto Final"() -> (w365:dbl)
                n103 = Greater Or Equal?(x=w365, y=w366) -> (x >= y?=w367:bool)
                n104 = case shown="True" w367 {
                  tunnel: w366 -> [w371 w374]
                  tunnel: [w371 w373] -> w369
                  tunnel: ["Setimo" "First"] -> w368
                  frame False {
                  }
                  frame True {
                    n105 = Multiply(x=0, y=w374) -> (x*y=w373:dbl)
                  }
                }
              }
              frame "Setimo" {
                n106 = And(x=w377, y=FALSE) -> (x .and. y?=w376:bool)
                n107 = case shown="True" w379 {
                  tunnel: w386 -> [_ w395]
                  tunnel: [0.0 w393] -> w380
                  tunnel: ["Setimo" "Terceiro"] -> w381
                  frame False {
                  }
                  frame True {
                    n108 = local read "Estoque \nProduto Final"() -> (w394:dbl)
                    n109 = Subtract(x=w394, y=w395) -> (x-y=w393:dbl)
                  }
                }
                n110 = Subtract(x=w385, y=w380) -> (x-y=w383:dbl)
                n111 = Subtract(x=w384, y=w380) -> (x-y=w382:dbl)
                n112 = local write "Estoque \nProduto A [KG]"(w383) -> ()
                n113 = local write "Estoque \nProduto B [KG]"(w382) -> ()
              }
              frame "First", Default {
                n114 = case shown="False" "Contagem de Estoque OK?" {
                  tunnel: [0.0 w428] -> w418
                  tunnel: [0.0 w427] -> w417
                  tunnel: w415 -> [_ w428]
                  tunnel: w414 -> [_ w427]
                  frame False {
                  }
                  frame True {
                  }
                }
                n115 = Add(x=w418, y=w422) -> (x+y=w420:dbl)
                "Estoque \nProduto A [KG]" <- w420
                n116 = Add(x=w421, y=w417) -> (x+y=w419:dbl)
                "Estoque \nProduto B [KG]" <- w419
                n117 = local read "Estoque \nProduto A [KG]"() -> (w408:dbl)
                n118 = local read "Estoque \nProduto B [KG]"() -> (w401:dbl)
                n119 = local read "Estoque \nProduto B [KG]"() -> (w403:dbl)
                n120 = local read "Estoque A utilizado:"() -> (w411:dbl)
                n121 = local read "Estoque B utilizado:"() -> (w400:dbl)
                n122 = Multiply(x=w408, y=0.5) -> (x*y=w404:dbl)
                n123 = Greater?(x=w408, y=w411) -> (0:w407:bool)
                n124 = Greater?(x=w401, y=w400) -> (0:w399:bool)
                n125 = Greater Or Equal?(x=w403, y=w404) -> (x >= y?=w402:bool)
                n126 = Or(x=w402, y=w399) -> (x .or. y?=w398:bool)
                n127 = And(x=w407, y=w398) -> (x .and. y?=w410:bool)
                n128 = case shown="True" w410 {
                  tunnel: ["First" "Second"] -> w416
                  frame False {
                  }
                  frame True {
                  }
                }
              }
              frame "Second" {
                n129 = Equal?(x=w433, y=TRUE) -> (x = y?=w444:bool)
                n130 = case shown="False" w444 {
                  tunnel: ["Second" "Entre"] -> w442
                  tunnel: [0.0 w454] -> w439
                  tunnel: w435 -> [_ w454]
                  tunnel: [0.0 w453] -> w441
                  tunnel: w434 -> [_ w453]
                  tunnel: [0.0 w452] -> w431
                  frame False {
                  }
                  frame True {
                    n131 = Add(x=w454, y=w453) -> (x+y=w452:dbl)
                  }
                }
                n132 = Subtract(x=w447, y=w441) -> (x-y=w445:dbl)
                n133 = Subtract(x=w440, y=w439) -> (x-y=w446:dbl)
                n134 = local write "Estoque \nProduto A [KG]"(w446) -> ()
                n135 = local write "Estoque \nProduto B [KG]"(w445) -> ()
                n136 = Add(x=w431, y=w432) -> (x+y=w430:dbl)
              }
            }
            "Thermometro\nForno" <- "Temperatura Desejada Forno °C"
          }
        }
        n137 = TCP Read(connection ID=w172, bytes to read=100, 7:T1."CRLF" ("mode (standard)"), 9:100 ("timeout ms (25000)")) -> (connection ID out=w176:refnum<k5>, data out=w171:string)  [unwired: 1 in, 1 out]
        "Protocolo de Ordens de Produção:" <- w171
        n138 = case shown="True" "Report:" {
          tunnel: [_ w502] -> w165
          frame False {
          }
          frame True {
            w482 = ","
            n139 = case shown="False" "Enviar" {
              tunnel: [w504 "Mensagem"] -> w502
              frame False {
                n140 = local read "Protocolo de Comunicação - Produção"() -> (w504:string)
              }
              frame True {
              }
            }
            n141 = local read "Estoque \nProduto A [KG]"() -> (w501:dbl)
            n142 = local read "Estoque \nProduto B [KG]"() -> (w500:dbl)
            n143 = local read "Estoque A utilizado:"() -> (w499:dbl)
            n144 = Number To Decimal String(number=w501) -> (decimal integer string=w496:string)  [unwired: 1 in]
            n145 = Number To Decimal String(number=w500) -> (decimal integer string=w495:string)  [unwired: 1 in]
            n146 = Number To Decimal String(number=w499) -> (decimal integer string=w494:string)  [unwired: 1 in]
            n147 = local read "Thermometro\nForno"() -> (w488:dbl)
            n148 = local read "LED Misturador"() -> (w486:bool)
            n149 = local read "Estoque B utilizado:"() -> (w498:dbl)
            n150 = Boolean To (0,1)(Boolean=w486) -> (0, 1=w485:i16)
            n151 = Number To Decimal String(number=w498) -> (decimal integer string=w493:string)  [unwired: 1 in]
            n152 = Number To Decimal String(number=w488) -> (decimal integer string=w492:string)  [unwired: 1 in]
            n153 = Number To Decimal String(number=w485) -> (decimal integer string=w487:string)  [unwired: 1 in]
            n154 = local read "Estoque \nProduto Final"() -> (w497:dbl)
            n155 = local read "LED Forno"() -> (w484:bool)
            n156 = Boolean To (0,1)(Boolean=w484) -> (0, 1=w483:i16)
            n157 = Number To Decimal String(number=w497) -> (decimal integer string=w490:string)  [unwired: 1 in]
            n158 = Number To Decimal String(number=w483) -> (decimal integer string=w491:string)  [unwired: 1 in]
            n159 = local read "Chave"() -> (w481:string)
            n160 = Concatenate Strings(w496, w482, w495, w482, w494, w482, w493, w482, w492, w482, w487, w482, w491, w482, w490, w482, w481) -> (→"Protocolo de Comunicação - Produção":string)
          }
        }
        n161 = String Length(string=w171) -> (length=w178:i32)
        n162 = formula code="if((EstA==0)&&(EstB==0)){\nchave = 9;\n};\n\nif((EstA>1)&&(EstA<50)&&(EstB>50)&&(temp>40)&&(temp<70)&&(Key==1)){\nchave = 1;\n};\n\nif((EstA==0)&&(EstB>50)&&(temp>40)&&(temp<70)&&(Key==1)){\nchave = 2;\n};\n\nif((EstB==0)&&(EstA>50)&&(temp>40)&&(temp<70)&&(Key==1)){\nchave = 4;\n};\n\nif((EstB>1)&&(EstB<50)&&(EstA>50)&&(temp>40)&&(temp<70)&&(Key==1)){\nchave = 3;\n};\n\nif((EstA>50)&&(EstB>50)&&(temp>40)&&(temp<70)&&(Key==1)){\nchave = 5;\n};\n\nif((temp<40)||(temp>70)&&(Key==1)){\nchave = 6;\n};\n\nif(Key==0){\nchave = 7;\n};\n\nif(Ped>EstA){\nchave = 8;\n};"("EstA"=w157, "EstB"=w156, "temp"=w155, "Key"=w153, "Ped"=w140) -> ("chave"=w147:dbl)
        n163 = Not Equal To 0?(x=w178) -> (x != 0?=w175:bool)
        n164 = local read "Estoque A utilizado:"() -> (w152:dbl)
        n165 = local read "Estoque \nProduto Final"() -> (w141:dbl)
        n166 = local read "Estoque B utilizado:"() -> (w151:dbl)
        n167 = case shown="False" w175 {
          tunnel: ["Enviar" "Espera"] -> w174
          frame False {
          }
          frame True {
          }
        }
        n168 = Add(x=w152, y=w151) -> (x+y=w149:dbl)
        n169 = To Long Integer(number=w147) -> (32bit integer=w136:i32)
        n170 = Greater Or Equal?(x=w141, y=w149) -> (x >= y?=w142:bool)
        n171 = Number To Decimal String(number=w136) -> (decimal integer string=→"Chave":string)  [unwired: 1 in]
        n172 = Greater Than 0?(x=w141) -> (x > 0?=w143:bool)
        n173 = And(x=w142, y=w143) -> (x .and. y?=w144:bool)
        n174 = Concatenate Strings(w165, "\r", "\n") -> (w184:string)
        n175 = case shown="9" w136 {
          tunnel: ["OK" "Estoque A no minimo" " Estoque A acabou" "Estoque B no minimo\n" "Estoque B acabou" "OK" "Temperatura Forno NOK" "Esteira Parada" "Pedido Superior ao Estoque" "Sem Estoque"] -> w146
          tunnel: [u32 6618880 ("Pedido") u32 15859456 ("Pedido") u32 16711680 ("Pedido") u32 15859456 ("Pedido") u32 16711680 ("Pedido") u32 6618880 ("Pedido") u32 16711680 ("Pedido") u32 16711680 ("Pedido") u32 15859456 ("Pedido") u32 16718848 ("Pedido")] -> w145
          frame 0, Default {
          }
          frame 1 {
          }
          frame 2 {
          }
          frame 3 {
          }
          frame 4 {
          }
          frame 5 {
          }
          frame 6 {
          }
          frame 7 {
          }
          frame 8 {
          }
          frame 9 {
          }
        }
        "Funcionamento:" <- w145
        "Funcionamento:" <- w146
        n176 = case shown="True" w144 {
          tunnel: [u32 15859456 ("Pedido") u32 6618880 ("Pedido")] -> w150
          tunnel: ["Pedido em Criação" "Pedido Pronto"] -> w148
          frame False {
          }
          frame True {
          }
        }
        "Pedido" <- w150
        "Pedido" <- w148
        n177 = TCP Write(connection ID=w176, data in=w184, 9:100 ("timeout ms (25000)")) -> (connection ID out=w187:refnum<k5>)  [unwired: 1 in, 2 out]
        n178 = case shown="True" "RESET \nDE SIMULA敲O" {
          frame False {
          }
          frame True {
            w480 = 0.0
            n179 = local write "Estoque \nProduto Final"(w480) -> ()
            n180 = local write "Estoque \nForno"(w480) -> ()
            n181 = local write "Thermometro\nForno"(w480) -> ()
            n182 = local write "Estoque \nProduto A [KG]"(w480) -> ()
            n183 = local write "Estoque \nProduto B [KG]"(w480) -> ()
            n184 = local write "Estoque \nMisturador"(w480) -> ()
            n185 = local write "Estoque Produto B"(w480) -> ()
            n186 = local write "Estoque A utilizado:"(w480) -> ()
            n187 = local write "Estoque Produto A"(w480) -> ()
            n188 = local write "Estoque B utilizado:"(w480) -> ()
            n189 = local write "Temperatura Desejada Forno °C"(w480) -> ()
          }
        }
        n190 = Wait (ms)(milliseconds to wait=u32 1000) -> ()  [unwired: 1 out]
      }
    }
  }
  n191 = TCP Close Connection(connection ID=w10) -> ()  [unwired: 2 in, 2 out]
